vi "TCP Server.vi"() -> ()   [LabVIEW 2020]
uses:
  <userlib>/_NEVSTOP/Communicable State Machine(CSM)/_Support/Typedef/_CSM_GlobalLog_MSG.ctl
  <userlib>/_NEVSTOP/Communicable State Machine(CSM)/_Support/Typedef/_CSM_Response Source Message.ctl
  <userlib>/_NEVSTOP/Communicable State Machine(CSM)/_Support/Typedef/_CSM_GlobalLog_MSG_TYPE.ctl
  <userlib>/_NEVSTOP/Communicable State Machine(CSM)/_Support/Priority Queue/Priority Queue.lvclass/Priority Queue.ctl
  931d4ba7-b454-410e-88bd-402e2cce69a9.vi
  <vilib>/Utility/error.llb/Clear Errors.vi
  <userlib>/_NEVSTOP/Communicable State Machine(CSM)/_Support/GlobalEvent/Gevt-ThreadQueueName.vi
  931d4ba7-b454-410e-88bd-402e2cce69a9.vi/b09b9099-6be0-413b-8afc-4908471460c3.vi
  <userlib>/_NEVSTOP/Communicable State Machine(CSM)/_Support/Process/CSMP-Sync Call.vi
  <userlib>/_NEVSTOP/Communicable State Machine(CSM)/Utility/uuid.vi
  <userlib>/_NEVSTOP/Communicable State Machine(CSM)/Utility/Build Error Cluster.vi
  <userlib>/_NEVSTOP/Communicable State Machine(CSM)/Utility/Trim Both Whitespace.vi
  <userlib>/_NEVSTOP/Communicable State Machine(CSM)/_Support/CSMQ/_CSMObj-Message Check.vi
  <userlib>/_NEVSTOP/Communicable State Machine(CSM)/_Support/CSMQ/_CSMObj-Enqueue Cross-Module Message.vi
  <userlib>/_NEVSTOP/Communicable State Machine(CSM)/_Support/CSMQ/_CSMOFGV Get.vi
  <userlib>/_NEVSTOP/Communicable State Machine(CSM)/_Support/Priority Queue/Enqueue Element.vi
  <userlib>/_NEVSTOP/Communicable State Machine(CSM)/addons/INI-Static-Variable-Support/_Support/global-csm-ini-db-change-flag.vi
  <vilib>/Utility/Data Type/Get Type Information.vi
  <userlib>/_NEVSTOP/Communicable State Machine(CSM)/addons/API-String-Arugments-Support/_Support/Data To SingleElementsArray_csm.vi
  <userlib>/_NEVSTOP/Communicable State Machine(CSM)/addons/INI-Static-Variable-Support/_Support/Parse Used Session and Name.vi
  <userlib>/_NEVSTOP/Communicable State Machine(CSM)/addons/API-String-Arugments-Support/_Support/Data To API String Arguments.vi
  <userlib>/_NEVSTOP/Communicable State Machine(CSM)/addons/INI-Static-Variable-Support/_Support/INI-FGV.vi
  <userlib>/_NEVSTOP/Communicable State Machine(CSM)/addons/API-String-Arugments-Support/_Support/Convert API String Arguments to Data(variant).vi
  <userlib>/_NEVSTOP/Communicable State Machine(CSM)/addons/API-String-Arugments-Support/_Support/SingleElementsArray To Data_csm.vi
  <userlib>/_NEVSTOP/Communicable State Machine(CSM)/_Support/FGV-BroadcastRegistry/global-CSMQ FGV Change Flag.vi
  <userlib>/_NEVSTOP/Communicable State Machine(CSM)/_Support/CSMQ/_CSMOFGV.vi
  <userlib>/_NEVSTOP/Communicable State Machine(CSM)/_Support/Error/CSM No Target Error.vi
  <userlib>/_NEVSTOP/Communicable State Machine(CSM)/_Support/Error/CSM Not Allowed Message.vi
  <userlib>/_NEVSTOP/Communicable State Machine(CSM)/_Support/Error/CSM Target Error.vi
  <userlib>/_NEVSTOP/Communicable State Machine(CSM)/_Support/Error/CSM Unhandled State Error.vi
  <userlib>/_NEVSTOP/Communicable State Machine(CSM)/_Support/Error/CSM Target Timeout Error.vi
  <vilib>/addons/_JKI.lib/_JKI_lib_TCP_Server.llb/JKI TCP Server.lvclass
  <userlib>/_NEVSTOP/Communicable State Machine(CSM)/Communicable State Machine.lvlib
panel:
  in  "stop":bool
  out "No. of Connections":u32
  out "Time Running":dbl[unit] format="%#.0p"
  in  "Disconnect all clients?":bool
  out "State History":string
  out "Connections Info":T1(array[cluster])
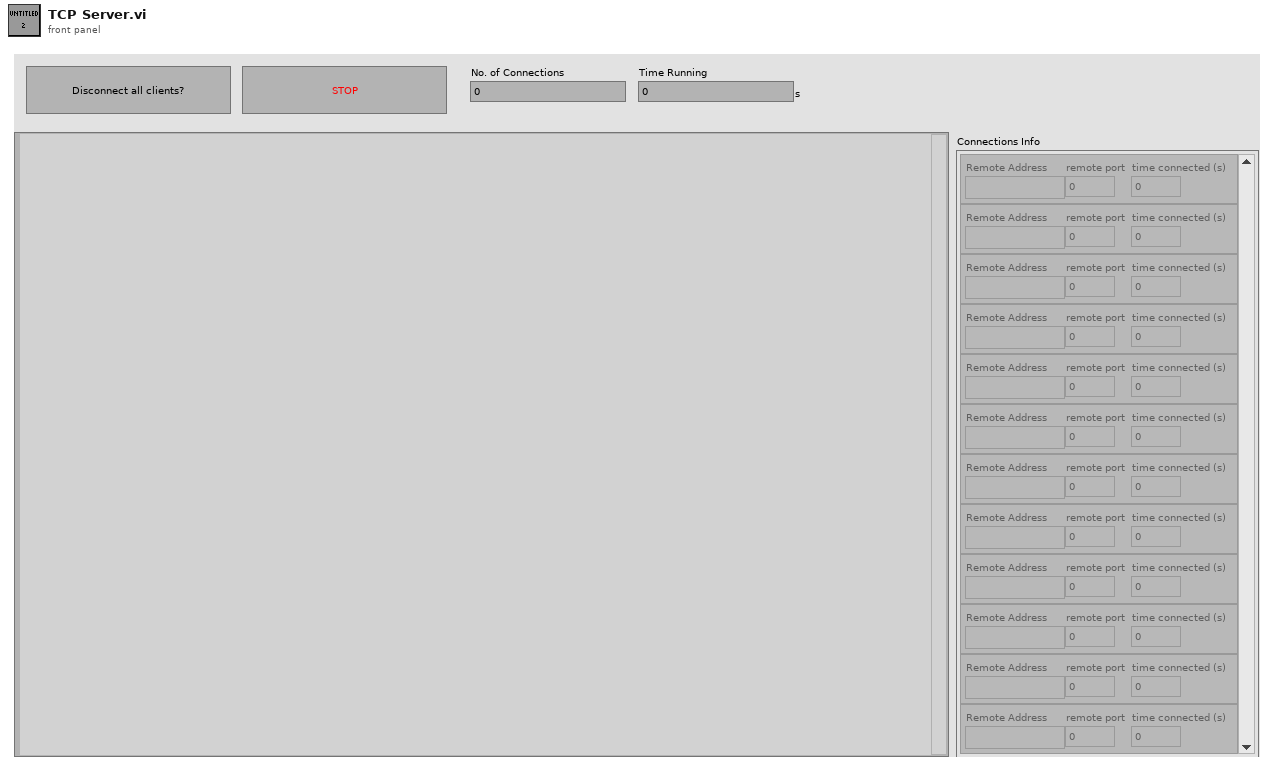
[diagram p1: front panel]
types:
  T1 = cluster{"Remote Address":string, "remote port":u16, "time connected (s)":dbl}[]
  T2 = cluster{"Server.Port":u16, "Server.MaxConnections":u32}
  T3 = cluster{"threashold(#/s)":dbl, "Check Peroid(s)":dbl}
  T4 = typedef "Communicable State Machine.lvlib/_CSM_GlobalLog_MSG.ctl" = cluster{"Name(\"\" to use uuid)":string, "Current State":string, "Arguments":string, "Source Message":T5, "Source Module":string, "Complete(T)/Start(F)":bool, "LogType":T6}
  T5 = typedef "Communicable State Machine.lvlib/_CSM_Response Source Message.ctl" = cluster{"‘State":string, "’Arguments":string, "’Error":errorcluster}
  T6 = typedef "Communicable State Machine.lvlib/_CSM_GlobalLog_MSG_TYPE.ctl" = enum16{"User Log", "State Change", "Status", "Interrupt", "Register", "Unregister", "Error Log", "Module Created", "Module Destroyed"}
  T7 = typedef "JKI TCP Server.lvclass/TCP Server Public Connections Info Cluster.ctl" = cluster{"Remote Address":string, "remote port":u16, "time connected (s)":dbl}
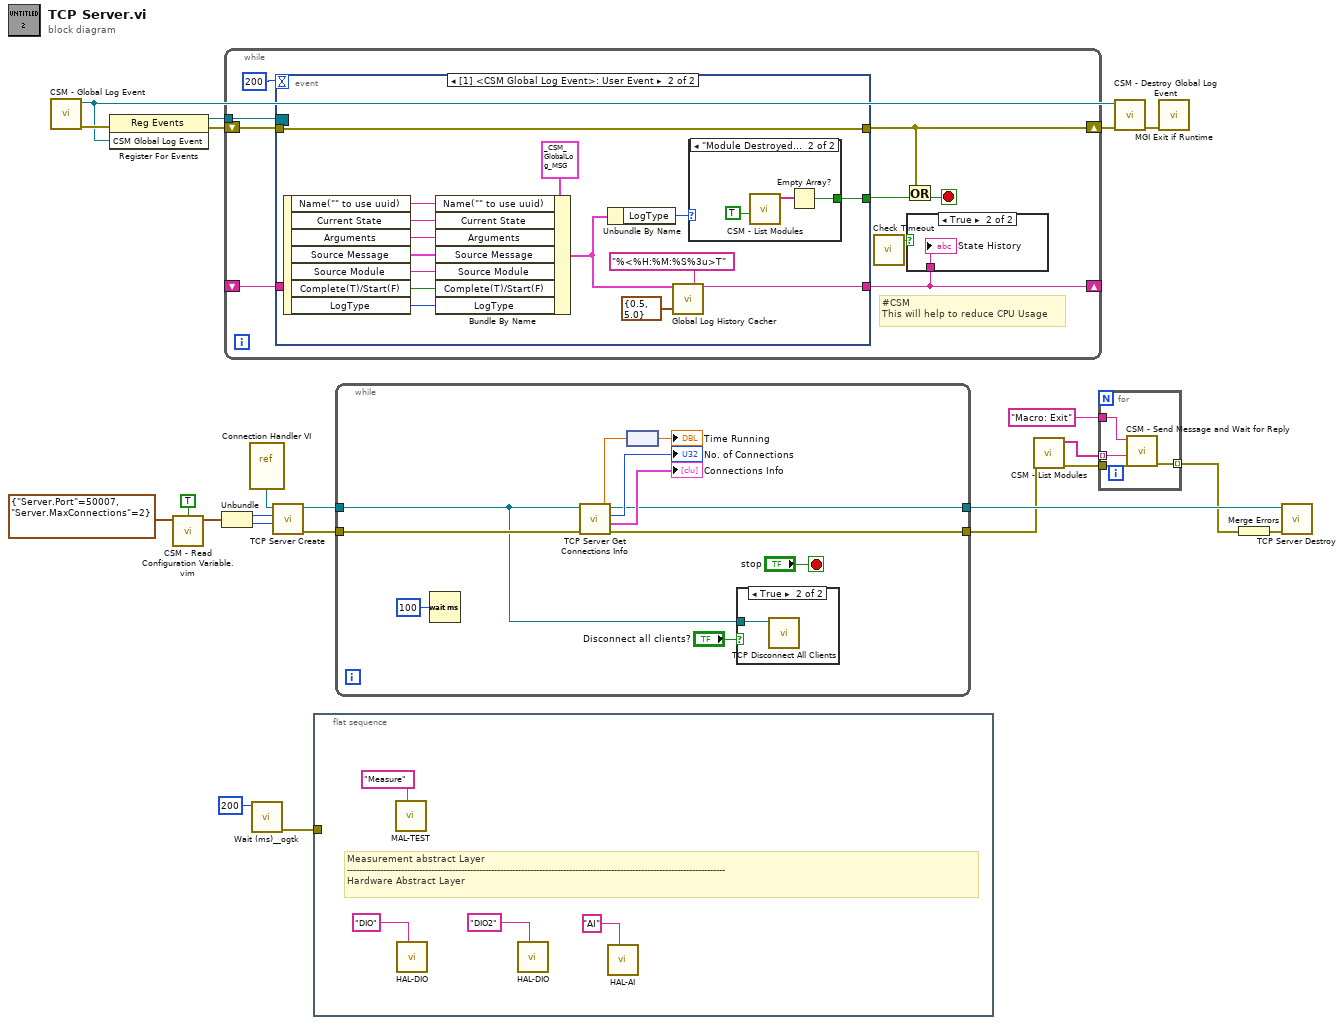
[diagram p0: block diagram]
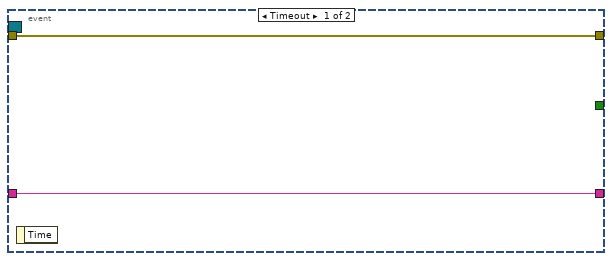
[diagram p4: hidden frame]
diagram:
  n1 = call <userlib>:"CSM - Global Log Event.vi"() -> ("Error out"=w6:errorcluster, "CSM Global Log Event"=w4:refnum<user-event>)  [unwired: 10 in]
  n2 = register-events(error in=w6, w4) -> (reference out=w7:refnum<event-registration>, error out=w8:errorcluster)  [unwired: 1 in]
  n3 = call "CSM - Read Configuration Variable.vim"("Write If not found?(F)"=TRUE, "config prototype(Cluster Prefered)"=T2 {"Server.Port"=50007, "Server.MaxConnections"=2}) -> ("config out"=w19:T2)  [unwired: 6 in, 1 out]
  n4 = Unbundle(w19) -> ("Server.Port"=w18:u16, "Server.MaxConnections"=w9:u32)
  n5 = while {
    tunnel: w7 -> [w32]
    shift-right: [w29] -> w5
    shift-left: w8 -> [w31]
    shift-right: [w26] -> _
    shift-left: _ -> [w25]
    stop <- w30 stop-if-true
    # "#CSM\nThis will help to reduce CPU Usage"
    n6 = event shown="[1] <CSM Global Log Event>: User Event" {
      selector: w32 -> [_ _]
      dyn-events: _ -> [_ _]
      timeout: 200 -> [_ _]
      tunnel: w31 -> [w35 w50]
      tunnel: [w35 w50] -> w29
      tunnel: [_ w39] -> w28
      tunnel: [w34 w36] -> w26
      tunnel: w25 -> [w34 _]
      event Timeout {
        n7 = event-data() -> ()  [unwired: 1 in, 1 out]
      }
      event User Event {
        n8 = event-data() -> ("Name(\"\" to use uuid)"=w49:string, "Current State"=w48:string, "Arguments"=w47:string, "Source Message"=w46:T5, "Source Module"=w45:string, "Complete(T)/Start(F)"=w44:bool, "LogType"=w43:T6)  [unwired: 1 in]
        n9 = Bundle By Name(cluster=T4 {"Name(\"\" to use uuid)"="", "Current State"="", "Arguments"="", "Source Message"={"‘State"="", "’Arguments"="", "’Error"={"status"=FALSE, "code"=0, "source"=""}}, "Source Module"="", "Complete(T)/Start(F)"=FALSE, "LogType"=enum."State Change"} ("Cross CSM Data"), "Name(\"\" to use uuid)"=w49, "Current State"=w48, "Arguments"=w47, "Source Message"=w46, "Source Module"=w45, "Complete(T)/Start(F)"=w44, "LogType"=w43) -> (w41:T4)
        n10 = Unbundle By Name(w41) -> ("LogType"=w40:T6)
        n11 = call <userlib>:"Global Log History Cacher.vi"("Cross CSM Data"=w41, "Time format string"="%<%H:%M:%S%3u>T", "Settings"=T3 {"threashold(#/s)"=0.5, "Check Peroid(s)"=5.0}) -> ("String Cache"=w36:string)  [unwired: 11 in, 1 out]
        n12 = case shown="\"Module Destroyed\"" w40 {
          tunnel: [_ w51] -> w39
          frame "User Log", Default {
          }
          frame "Module Destroyed" {
            n13 = call <userlib>:"CSM - List Modules.vi"("All?"=TRUE) -> ("Module Names"=w53:string[])  [unwired: 9 in, 1 out]
            n14 = Empty Array?(array=w53) -> (empty?=w51:bool)
          }
        }
      }
    }
    n15 = call <userlib>:"Check Timeout.vi"() -> ("Timeout"=w24:bool)  [unwired: 8 in]
    n16 = Or(x=w29, y=w28) -> (x .or. y?=w30:bool)
    n17 = case shown="True" w24 {
      tunnel: w26 -> [_ w33]
      frame False {
      }
      frame True {
        "State History" <- w33
      }
    }
  }
  n18 = vi-ref "Connection Handler VI.vi"() -> ("vi reference"=w10:refnum<vi>)
  n19 = call <userlib>:"Wait (ms)__ogtk.vi"("milliseconds to wait"=u32 200) -> ("error out"=w3:errorcluster)  [unwired: 9 in, 1 out]
  n20 = call <vilib>:"TCP Server Create.vi"("max connections (0: no limit)"=w9, "port"=w18, "Connection Handler Call-Back VI RefNum"=w10) -> ("error out"=w23:errorcluster, "TCP Server"=w22:refnum<class "JKI TCP Server.lvclass">)  [unwired: 7 in]
  n21 = flat-sequence {
    tunnel: w3 -> [_]
    frame #0 {
      # "Measurement abstract Layer\n------------------------------------------------------------------------------------------------------------------------------\nHardware Abstract Layer"
      n22 = call "MAL-TEST.vi"("Name(\"\" to use uuid)"="Measure" ("Name(\"\" to use uuid)")) -> ()  [unwired: 11 in]
      n23 = call "HAL-DIO.vi"("Name(\"\" to use uuid)"="DIO" ("Name(\"\" to use uuid)")) -> ()  [unwired: 11 in]
      n24 = call "HAL-DIO.vi"("Name(\"\" to use uuid)"="DIO2" ("Name(\"\" to use uuid)")) -> ()  [unwired: 11 in]
      n25 = call "HAL-AI.vi"("Name(\"\" to use uuid)"="AI" ("Name(\"\" to use uuid)")) -> ()  [unwired: 11 in]
    }
  }
  n26 = while {
    tunnel: w23 -> [w63]
    tunnel: w22 -> [w60]
    tunnel: [w62] -> w21
    tunnel: [w61] -> w16
    stop <- "stop" stop-if-true
    n27 = Wait (ms)(milliseconds to wait=u32 100) -> ()  [unwired: 1 out]
    n28 = call <vilib>:"TCP Server Get Connections Info.vi"("error in (no error)"=w63, "TCP Server"=w60) -> ("error out"=w61:errorcluster, "Connections Info"=→"Connections Info":T7[], "Number of Connections"=→"No. of Connections":u32, "TCP Server out"=w62:refnum<class "JKI TCP Server.lvclass">, "time running (s)"=w66:dbl)  [unwired: 5 in]
    n29 = node(w66) -> (→"Time Running":dbl[unit])
    n30 = case shown="True" "Disconnect all clients?" {
      tunnel: w60 -> [_ w69]
      frame False {
      }
      frame True {
        n31 = call <vilib>:"TCP Disconnect All Clients.vi"("TCP Server"=w69) -> ()  [unwired: 9 in, 2 out]
      }
    }
  }
  n32 = call <userlib>:"CSM - List Modules.vi"("Error in"=w16) -> ("Error out"=w15:errorcluster, "Module Names"=w14:string[])  [unwired: 9 in]
  n33 = for {
    tunnel: w15 -> [w73]
    tunnel: w14 -> [w72] mode=indexing
    tunnel: "Macro: Exit" ("State") -> [w71]
    tunnel: [w70] -> w12 mode=indexing
    n34 = call <userlib>:"CSM - Send Message and Wait for Reply.vi"("Error In (no error)"=w73, "Target Module"=w72, "State"=w71) -> ("error out"=w70:errorcluster)  [unwired: 6 in, 2 out]
  }
  n35 = call <userlib>:"CSM - Destroy Global Log Event.vi"("Error in"=w5, "CSM Global Log Event"=w4) -> ("Error out"=w1:errorcluster)  [unwired: 9 in]
  n36 = call <userlib>:"MGI Exit if Runtime.vi"("Error In (Dependency Only)"=w1) -> ()  [unwired: 11 in]
  n37 = Merge Errors(w12) -> (w17:errorcluster)
  n38 = call <vilib>:"TCP Server Destroy.vi"("error in (no error)"=w17, "TCP Server"=w21) -> ()  [unwired: 9 in, 1 out]
